vi "upgrade to websocket.vi"(8 "error in":errorcluster, 10 "upgrade data":T1, 11 "websocket handler in":refnum<class "websocket upgrade handler.lvclass">) -> (0 "error out":errorcluster)   [LabVIEW 2013, in "websocket upgrade handler.lvclass"]
uses:
  websocket upgrade handler.lvclass
  HTTP responder/http upgrade data.ctl
  http request.ctl
  http method.ctl
  websocket upgrade handler.lvclass/websocket upgrade handler.ctl
  user plugin/websocket user plugin.lvclass
  HTTP responder/http responder.lvclass
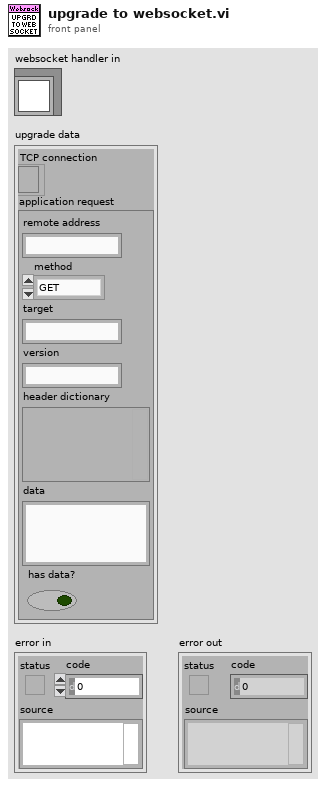
[diagram p1: front panel]
types:
  T1 = typedef "http responder.lvclass/http upgrade data.ctl" = cluster{"TCP connection":refnum<k5>, "application request":T2}
  T2 = typedef "http request.ctl" = cluster{"remote address":string, "method":T3, "target":string, "version":string, "header dictionary":variant, "data":string, "has data?":bool}
  T3 = typedef "http method.ctl" = enum16{"GET", "POST", "PUT", "DELETE", "HEAD", "OPTIONS", "upgrade"}
  T4 = typedef "websocket upgrade handler.lvclass/first byte header.ctl" = cluster{"fin":bool, "RSRV1":bool, "RSRV2":bool, "RSRV3":bool, "opcode":u8}
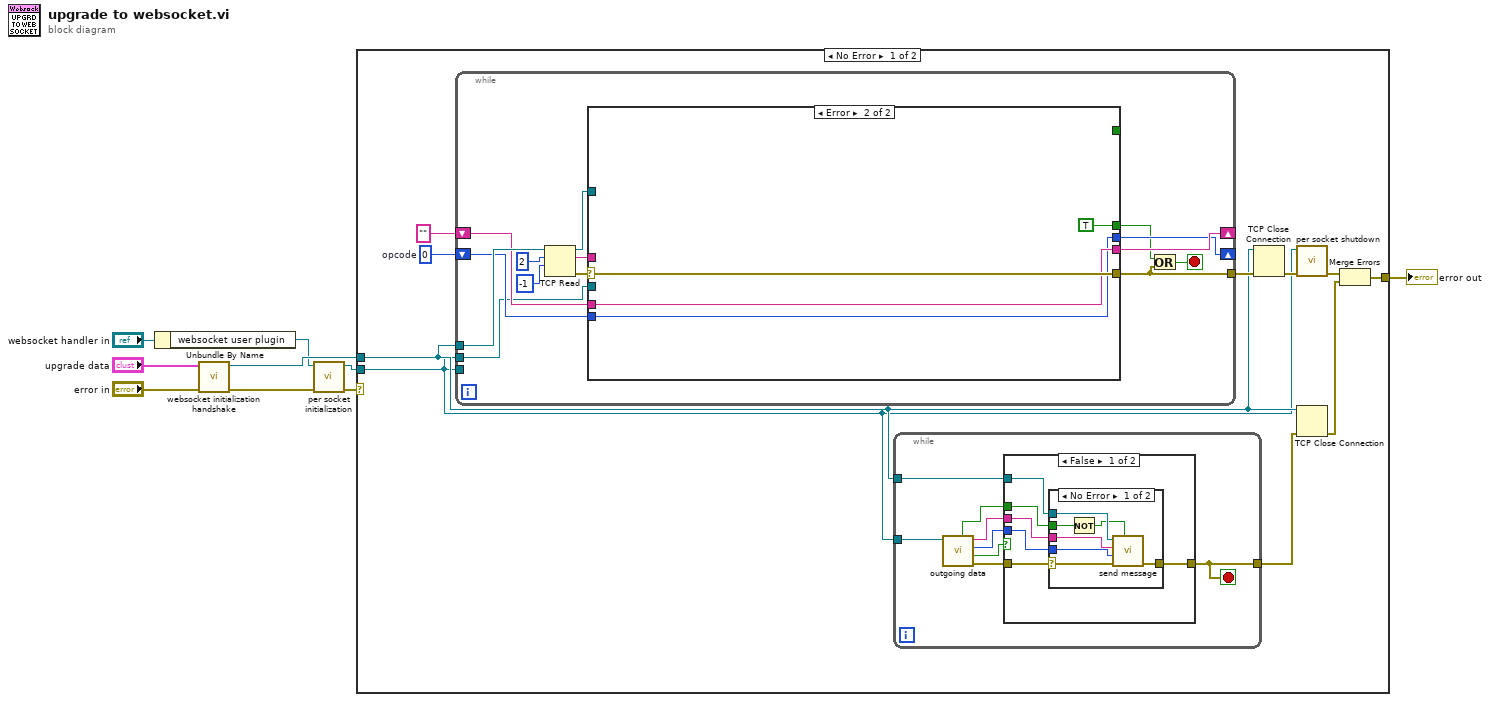
[diagram p0: block diagram]
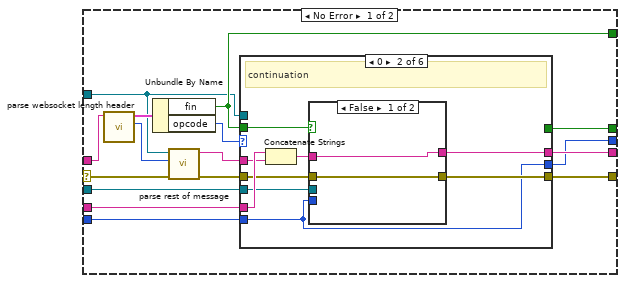
[diagram p4: hidden frame]
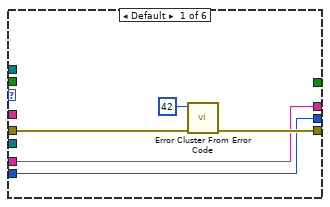
[diagram p5: hidden frame]
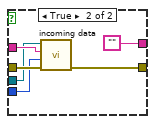
[diagram p6: hidden frame]
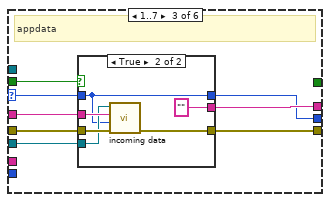
[diagram p7: hidden frame]
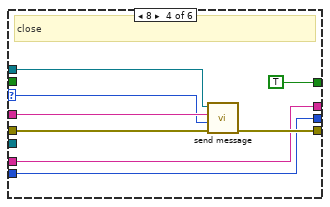
[diagram p9: hidden frame]
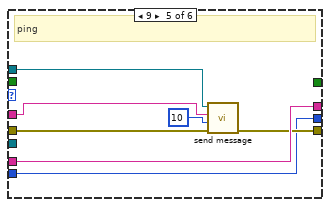
[diagram p10: hidden frame]
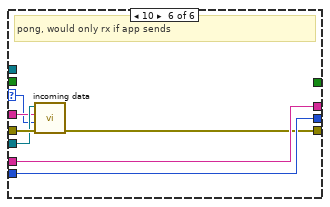
[diagram p11: hidden frame]
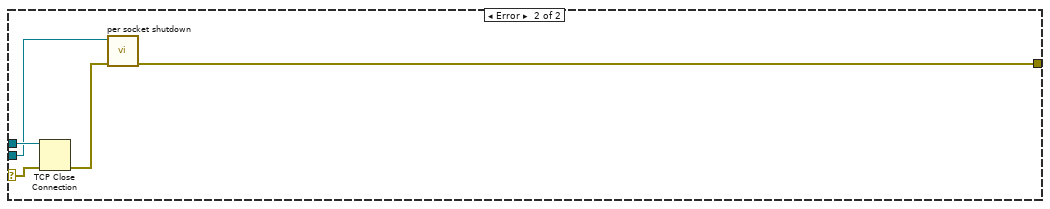
[diagram p12: hidden frame]
diagram:
  n1 = Unbundle By Name("websocket handler in") -> ("websocket user plugin"=w4:refnum<class "websocket user plugin.lvclass">)
  n2 = call "websocket initialization handshake.vi"("error in"="error in", "upgrade data"="upgrade data") -> ("error out"=w2:errorcluster, "TCP Network Connection out"=w9:refnum<k5>)  [unwired: 8 in]
  n3 = call-dynamic "per socket initialization.vi"("error in"=w2, "websocket user plugin in"=w4) -> ("error out"=w1:errorcluster, "websocket user plugin out"=w3:refnum<class "websocket user plugin.lvclass">)  [unwired: 8 in]
  n4 = case shown="No Error" w1 {
    selector: w1 -> [_ w141]
    tunnel: w9 -> [w11 w142]
    tunnel: [w13 w139] -> w6
    tunnel: w3 -> [w10 w138]
    frame No Error {
      w16 = u8 0  # opcode
      n5 = while {
        tunnel: w11 -> [w53]
        tunnel: [w50] -> w14
        tunnel: w10 -> [_]
        shift-right: [w48] -> _
        shift-left: "" -> [w49]
        shift-right: [w46] -> _
        shift-left: w16 -> [w47]
        tunnel: w10 -> [w45]
        stop <- w44 stop-if-true
        n6 = TCP Read(connection ID=w53, bytes to read=2, 9:-1 ("timeout ms (25000)")) -> (connection ID out=w54:refnum<k5>, data out=w56:string, error out=w52:errorcluster)  [unwired: 2 in]
        n7 = case shown="Error" w52 {
          selector: w52 -> [w72 w137]
          tunnel: w56 -> [w71 _]
          tunnel: w54 -> [w60 _]
          tunnel: [w68 w137] -> w50
          tunnel: w49 -> [w64 w136]
          tunnel: [w65 w136] -> w48
          tunnel: [w62 _] -> _
          tunnel: w47 -> [w57 w135]
          tunnel: [w58 w135] -> w46
          tunnel: w45 -> [w61 _]
          tunnel: [w59 TRUE] -> w43
          frame No Error {
            n8 = call "parse websocket length header.vi"("header string"=w71) -> ("length"=w70:u8, "first byte"=w69:T4)  [unwired: 9 in]
            n9 = Unbundle By Name(w69) -> ("fin"=w62:bool, "opcode"=w66:u8)
            n10 = call "parse rest of message.vi"("error in (no error)"=w72, "length"=w70, "TCP Network Connection in"=w60) -> ("error out"=w67:errorcluster, "unmasked data"=w63:string)  [unwired: 7 in]
            n11 = case shown="0" w66 {
              selector: w66 -> [_ _ w96 w114 _ w127]
              tunnel: [w76 w84 w102 w116 w121 w131] -> w68
              tunnel: w67 -> [w77 w83 w101 w117 w125 w130]
              tunnel: [w74 w80 w98 w113 w126 w133] -> w65
              tunnel: w64 -> [w74 w86 _ w113 w126 w133]
              tunnel: w63 -> [_ w85 w99 w119 w123 w128]
              tunnel: w62 -> [_ w82 w100 _ _ _]
              tunnel: w61 -> [_ w79 w97 _ _ w129]
              tunnel: w60 -> [_ _ _ w118 w122 _]
              tunnel: [_ _ _ TRUE _ _] -> w59
              tunnel: [w73 w78 w95 w112 w120 w132] -> w58
              tunnel: w57 -> [w73 w78 _ w112 w120 w132]
              frame Default {
                n12 = call <vilib>:"Error Cluster From Error Code.vi"("error in (no error)"=w77, "error code (0)"=42) -> ("error out"=w76:errorcluster)  [unwired: 7 in]
              }
              frame 0 {
                # "continuation"
                n13 = Concatenate Strings(w86, w85) -> (w81:string)
                n14 = case shown="False" w82 {
                  tunnel: [w88 w94] -> w84
                  tunnel: w83 -> [w88 w93]
                  tunnel: w81 -> [w87 w92]
                  tunnel: [w87 ""] -> w80
                  tunnel: w79 -> [_ w90]
                  tunnel: w78 -> [_ w89]
                  frame False {
                  }
                  frame True {
                    n15 = call-dynamic "incoming data.vi"("error in"=w93, "opcode"=w89, "data"=w92, "websocket user plugin in"=w90) -> ("error out"=w94:errorcluster)  [unwired: 7 in]
                  }
                }
              }
              frame 1..7 {
                # "appdata"
                n16 = case shown="True" w100 {
                  tunnel: [w105 w111] -> w102
                  tunnel: w101 -> [w105 w110]
                  tunnel: w99 -> [w104 w109]
                  tunnel: [w104 ""] -> w98
                  tunnel: w97 -> [_ w107]
                  tunnel: w96 -> [w103 w106]
                  tunnel: [w103 w106] -> w95
                  frame False {
                  }
                  frame True {
                    n17 = call-dynamic "incoming data.vi"("error in"=w110, "opcode"=w106, "data"=w109, "websocket user plugin in"=w107) -> ("error out"=w111:errorcluster)  [unwired: 7 in]
                  }
                }
              }
              frame 8 {
                # "close"
                n18 = call "send message.vi"("error in"=w117, "opcode"=w114, "data"=w119, "TCP Network Connection in"=w118) -> ("error out"=w116:errorcluster)  [unwired: 7 in]
              }
              frame 9 {
                # "ping"
                n19 = call "send message.vi"("error in"=w125, "opcode"=u8 10, "data"=w123, "TCP Network Connection in"=w122) -> ("error out"=w121:errorcluster)  [unwired: 7 in]
              }
              frame 10 {
                # "pong, would only rx if app sends"
                n20 = call-dynamic "incoming data.vi"("error in"=w130, "opcode"=w127, "data"=w128, "websocket user plugin in"=w129) -> ("error out"=w131:errorcluster)  [unwired: 7 in]
              }
            }
          }
          frame Error {
          }
        }
        n21 = Or(x=w43, y=w50) -> (x .or. y?=w44:bool)
      }
      n22 = while {
        tunnel: w11 -> [w27]
        tunnel: [w26] -> w15
        tunnel: w10 -> [w25]
        stop <- w26 stop-if-true
        n23 = call-dynamic "outgoing data.vi"("websocket user plugin in"=w25) -> ("error out"=w24:errorcluster, "timeout"=w20:bool, "opcode"=w21:u8, "data"=w22:string, "not last fragment (F)"=w23:bool)  [unwired: 6 in]
        n24 = case shown="False" w20 {
          tunnel: w27 -> [w33 _]
          tunnel: [w32 w42] -> w26
          tunnel: w24 -> [w31 w42]
          tunnel: w23 -> [w30 _]
          tunnel: w22 -> [w29 _]
          tunnel: w21 -> [w28 _]
          frame False {
            n25 = case shown="No Error" w31 {
              selector: w31 -> [w39 w41]
              tunnel: [w40 w41] -> w32
              tunnel: w33 -> [w38 _]
              tunnel: w30 -> [w37 _]
              tunnel: w29 -> [w35 _]
              tunnel: w28 -> [w34 _]
              frame No Error {
                n26 = Not(x=w37) -> (.not. x?=w36:bool)
                n27 = call "send message.vi"("final fragment (T)"=w36, "error in"=w39, "opcode"=w34, "data"=w35, "TCP Network Connection in"=w38) -> ("error out"=w40:errorcluster)  [unwired: 6 in]
              }
              frame Error {
              }
            }
          }
          frame True {
          }
        }
      }
      n28 = TCP Close Connection(connection ID=w11, error in (no error)=w14) -> (error out=w19:errorcluster)  [unwired: 1 in, 1 out]
      n29 = call-dynamic "per socket shutdown.vi"("error in (no error)"=w19, "websocket user plugin in"=w10) -> ("error out"=w18:errorcluster)  [unwired: 9 in]
      n30 = TCP Close Connection(connection ID=w11, error in (no error)=w15) -> (error out=w12:errorcluster)  [unwired: 1 in, 1 out]
      n31 = Merge Errors(w18, w12) -> (w13:errorcluster)
    }
    frame Error {
      n32 = TCP Close Connection(connection ID=w142, error in (no error)=w141) -> (error out=w140:errorcluster)  [unwired: 1 in, 1 out]
      n33 = call-dynamic "per socket shutdown.vi"("error in (no error)"=w140, "websocket user plugin in"=w138) -> ("error out"=w139:errorcluster)  [unwired: 9 in]
    }
  }
  "error out" <- w6
